vi "Framework Page.vi"(8 "error in (no error)":errorcluster, 11 "Node Ptr":T1 format="%.0x") -> (0 "error out":errorcluster)   [LabVIEW 2017, in "DSF System Explorer.lvlib"]
uses:
  DSF System Explorer.lvlib
  <vilib>/NI Veristand/Custom Device API/Custom Device Item Ref.ctl
  <vilib>/NI Veristand/Custom Device API/Custom Device API.lvlib
  Shared/DSF Shared.lvlib
  Data Viewer.lvlibp
panel:
  in  "New":bool
  in  "Version":string
  in  "Export":bool
  in  "Debug Mode":bool
  in  "Launch Data Viewer":bool
  in  "Server Frequency":dbl=20.0 format="%.0f Hz"
  in  "Enable Data Server":bool
  in  "Show Dialog on Error":bool
  in  "Show Threads":bool
  in  "Infinite FIFO Timeouts":bool
  in  "Measure Durations":bool
  in  "Measure Period":bool
  in  "Import":bool
  in  "View Configuration":bool
  in  "Header":cluster{"Section Name":string}={"Section Name"="Data Sharing Framework"}
  # "Debug Options"
  # "Measurement Options"
  # "Data Server Options"
  # "All Targets"
  # "All Targets"
  # "All Targets"
  # "Windows Only"
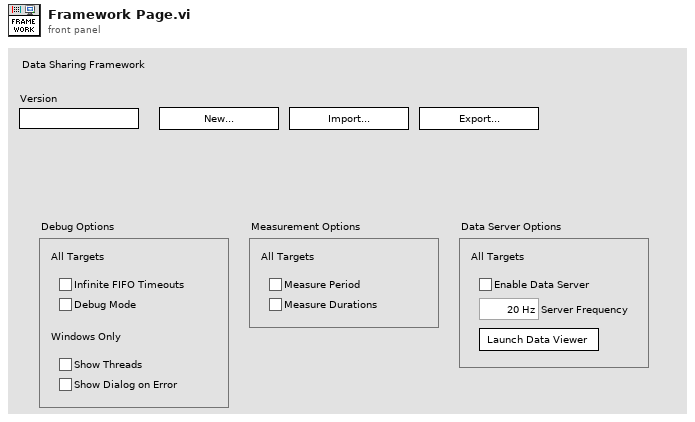
[diagram p1: front panel]
types:
  T1 = typedef "Custom Device API.lvlib/Custom Device Item Ref.ctl" = u64
  T2 = typedef "DSF Core.lvlibp/Framework.lvclass/Framework Options.ctl" = cluster{"FIFO Options":T3, "Thread Options":T4, "Plugin Options":T5, "Performance Options":T6, "Data Server Options":T7}
  T3 = typedef "DSF Core.lvlibp/Framework.lvclass/DSF FIFO Options.ctl" = cluster{"Infinite Timeouts":bool}
  T4 = typedef "DSF Core.lvlibp/Thread.lvclass/Thread Options.ctl" = cluster{"Show FP On Call":bool, "Close FP After Call":bool, "Allow Debugging":bool}
  T5 = typedef "DSF Core.lvlibp/Framework.lvclass/DSF Plugin Options.ctl" = cluster{"Default Components":bool}
  T6 = typedef "DSF Core.lvlibp/DSF Performance Options.ctl" = cluster{"Measure Period":bool, "Measure Rx/Tx Duration":bool}
  T7 = typedef "DSF Core.lvlibp/Framework.lvclass/Data Server Options.ctl" = cluster{"Enable Data Server":bool, "Period":u32}
  T8 = typedef "DSF Core.lvlibp/DSF Version Info.ctl" = cluster{"major":u32, "minor":u32, "fix":u32, "build":string}
  T9 = typedef "Custom Device API.lvlib/Custom Device Commands.ctl" = enum16{"Default", "Item renamed", "Shutdown", "Dynamic button pressed"}
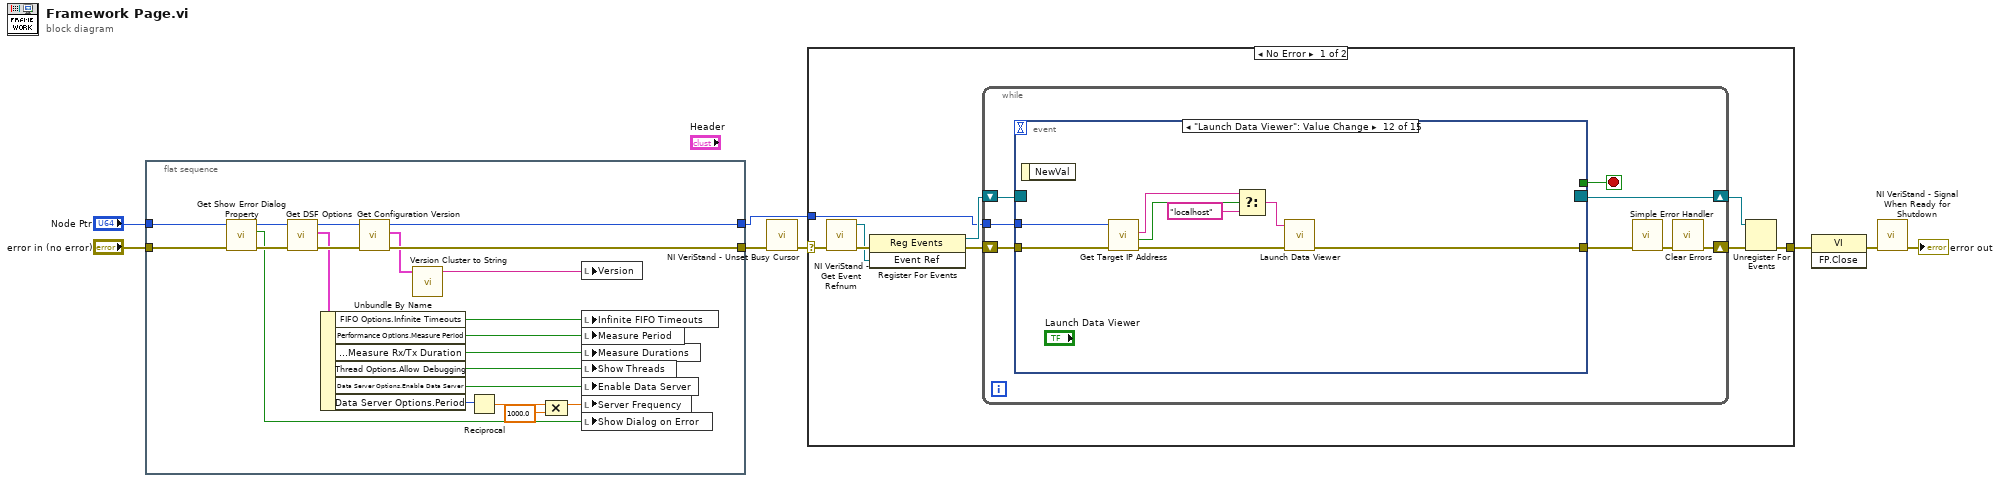
[diagram p0: block diagram]
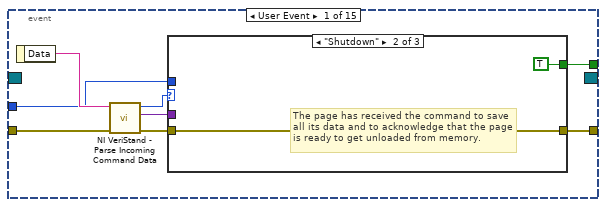
[diagram p2: hidden frame]
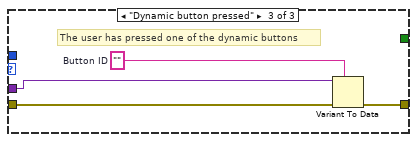
[diagram p4: hidden frame]
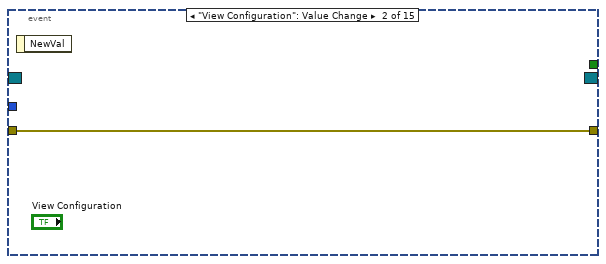
[diagram p5: hidden frame]
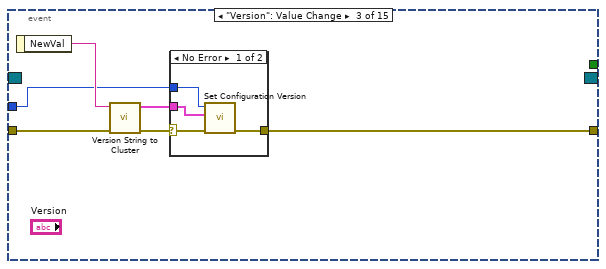
[diagram p6: hidden frame]
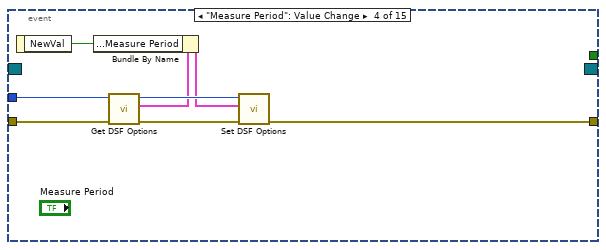
[diagram p8: hidden frame]
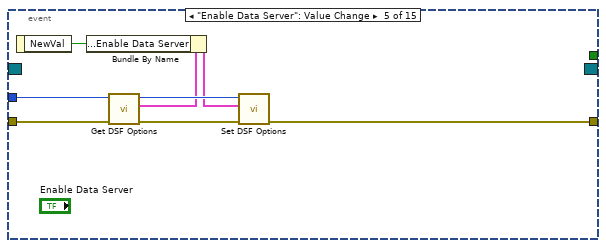
[diagram p9: hidden frame]
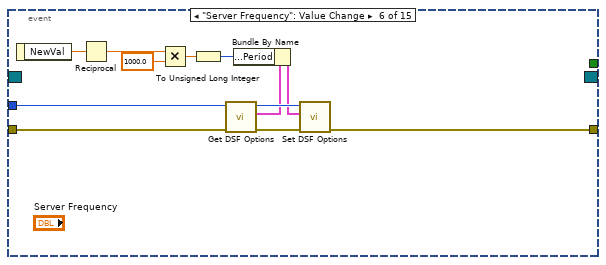
[diagram p10: hidden frame]
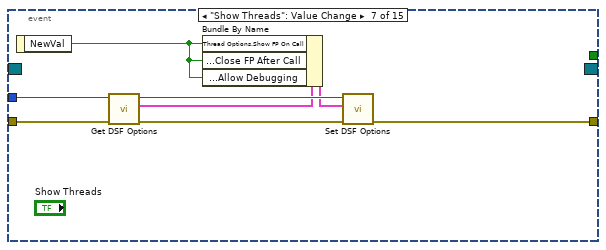
[diagram p11: hidden frame]
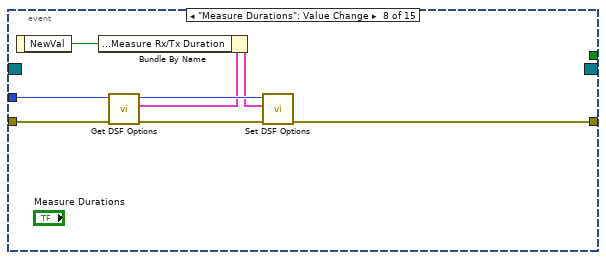
[diagram p12: hidden frame]
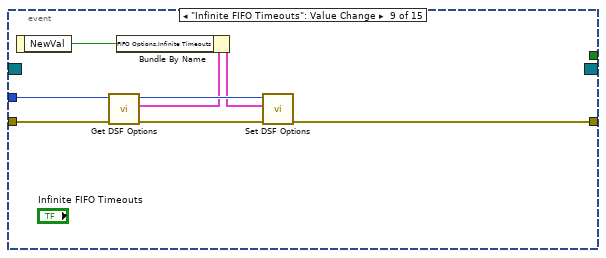
[diagram p13: hidden frame]
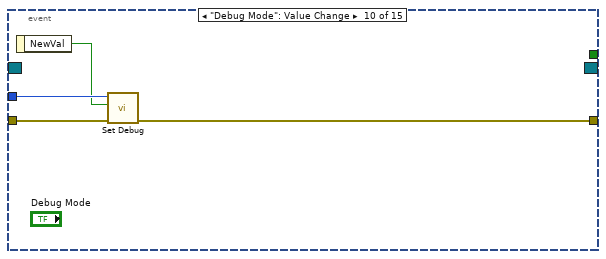
[diagram p14: hidden frame]
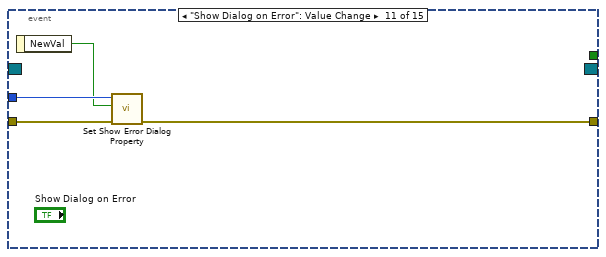
[diagram p15: hidden frame]
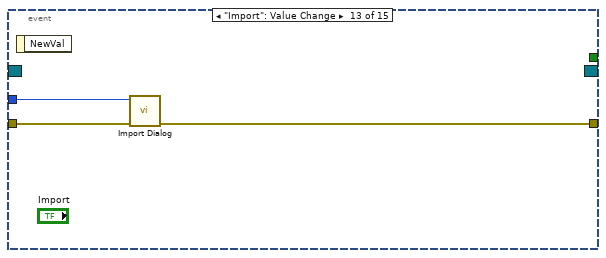
[diagram p16: hidden frame]
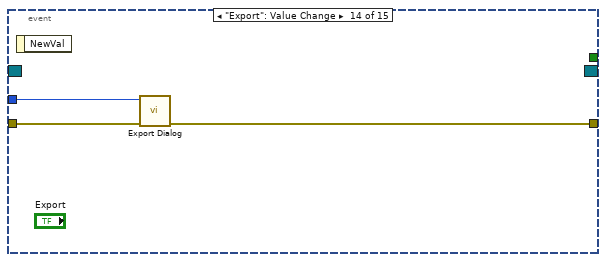
[diagram p17: hidden frame]
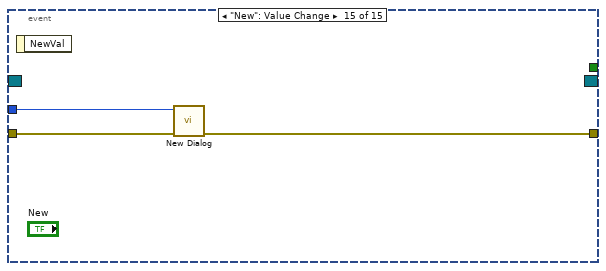
[diagram p18: hidden frame]
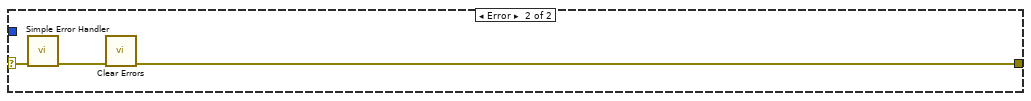
[diagram p19: hidden frame]
diagram:
  n1 = flat-sequence "Initialization code" {
    tunnel: "error in (no error)" -> [w9]
    tunnel: "Node Ptr" -> [w10]
    tunnel: [w14] -> w4
    tunnel: [w13] -> w1
    frame #0 {
      n2 = call "Get Show Error Dialog Property.vi"("error in (no error)"=w9, "Item Ref in"=w10) -> ("error out"=w24:errorcluster, "show error dialog"=w18:bool, "Item Ref out"=w25:T1)  [unwired: 7 in]
      n3 = call "Get DSF Options.vi"("error in (no error)"=w24, "Item Ref in"=w25) -> ("error out"=w17:errorcluster, "options"=w15:T2, "Item Ref out"=w16:T1)  [unwired: 7 in]
      n4 = Unbundle By Name(w15) -> ("FIFO Options.Infinite Timeouts"=w29:bool, "Performance Options.Measure Period"=w28:bool, "Performance Options.Measure Rx/Tx Duration"=w27:bool, "Thread Options.Allow Debugging"=w26:bool, "Data Server Options.Enable Data Server"=w23:bool, "Data Server Options.Period"=w22:u32)
      n5 = call "Get Configuration Version.vi"("error in (no error)"=w17, "Item Ref in"=w16) -> ("error out"=w14:errorcluster, "version"=w12:T8, "Item Ref out"=w13:T1)  [unwired: 7 in]
      n6 = call "Version Cluster to String.vi"("version"=w12) -> ("version string"=w11:string)  [unwired: 9 in, 1 out]
      n7 = Reciprocal(x=w22) -> (1/x=w21:dbl)
      n8 = Compound Arithmetic op=MULTIPLY(w21, 1000.0 ("y")) -> (w20:dbl)
      n9 = local write "Version"(w11) -> ()
      n10 = local write "Infinite FIFO Timeouts"(w29) -> ()
      n11 = local write "Measure Period"(w28) -> ()
      n12 = local write "Measure Durations"(w27) -> ()
      n13 = local write "Show Threads"(w26) -> ()
      n14 = local write "Enable Data Server"(w23) -> ()
      n15 = local write "Server Frequency"(w20) -> ()
      n16 = local write "Show Dialog on Error"(w18) -> ()
    }
  }
  n17 = call <vilib>:"NI VeriStand - Unset Busy Cursor.vi"("error in (no error)"=w4) -> ("error out"=w3:errorcluster)  [unwired: 10 out]
  n18 = case shown="No Error" w3 {
    selector: w3 -> [w30 w153]
    tunnel: [w35 w151] -> w8
    tunnel: w1 -> [w31 _]
    frame No Error {
      n19 = call <vilib>:"NI VeriStand - Get Event Refnum.vi"("error in (no error)"=w30) -> ("error out"=w38:errorcluster, "Event Ref"=w34:refnum<user-event>)  [unwired: 9 out]
      n20 = register-events(error in=w38, w34) -> (reference out=w32:refnum<event-registration>, error out=w33:errorcluster)  [unwired: 1 in]
      n21 = while {
        tunnel: w31 -> [w42]
        shift-right: [w39] -> w36
        shift-left: w33 -> [w45]
        shift-right: [w46] -> w37
        shift-left: w32 -> [w44]
        stop <- w43 stop-if-true
        n22 = event shown="[11] \"Launch Data Viewer\": Value Change" {
          selector: w44 -> [_ _ _ _ _ _ _ _ _ _ _ _ _ _ _]
          dyn-events: [_ _ _ _ _ _ _ _ _ _ _ _ _ _ _] -> w46
          timeout: _ -> [_ _ _ _ _ _ _ _ _ _ _ _ _ _ _]
          tunnel: w45 -> [w54 w62 w68 w79 w87 w100 w108 w115 w123 w129 w133 w141 w144 w147 w150]
          tunnel: [w50 _ _ _ _ _ _ _ _ _ _ _ _ _ _] -> w43
          tunnel: [w49 w62 w65 w76 w84 w98 w105 w112 w120 w126 w131 w138 w142 w145 w148] -> w41
          tunnel: w42 -> [w48 _ w63 w81 w89 w101 w109 w117 w125 w128 w132 w140 w143 w146 w149]
          event User Event {
            n23 = event-data() -> ("Data"=w53:string)  [unwired: 1 out]
            n24 = call <vilib>:"NI VeriStand - Parse Incoming Command Data.vi"("error in (no error)"=w54, "Incoming data"=w53) -> ("error out"=w52:errorcluster, "Outgoing data"=w47:variant, "Action"=w51:T9)  [unwired: 7 out]
            n25 = case shown="\"Shutdown\"" w51 {
              tunnel: w52 -> [w55 w56 w61]
              tunnel: [_ TRUE _] -> w50
              tunnel: [w55 w56 w58] -> w49
              tunnel: w48 -> [_ _ _]
              tunnel: w47 -> [_ _ w60]
              frame "Default", Default {
              }
              frame "Shutdown" {
                # "The page has received the command to save all its data and to acknowledge that the page is ready to get unloaded from memory."
              }
              frame "Dynamic button pressed" {
                w59 = ""  # Button ID
                # "The user has pressed one of the dynamic buttons"
                n26 = Variant To Data(error in=w61, type=w59, Variant=w60) -> (error out=w58:errorcluster)  [unwired: 1 out]
              }
            }
          }
          event "View Configuration": Value Change {
            n27 = event-data() -> ()  [unwired: 2 out]
          }
          event "Version": Value Change {
            n28 = event-data() -> ("NewVal"=w67:string)  [unwired: 1 out]
            n29 = call "Version String to Cluster.vi"("error in (no error)"=w68, "version string"=w67) -> ("error out"=w66:errorcluster, "version"=w64:T8)  [unwired: 8 in]
            n30 = case shown="No Error" w66 {
              selector: w66 -> [w72 w73]
              tunnel: [w69 w73] -> w65
              tunnel: w64 -> [w71 _]
              tunnel: w63 -> [w70 _]
              frame No Error {
                n31 = call "Set Configuration Version.vi"("error in (no error)"=w72, "version"=w71, "Item Ref in"=w70) -> ("error out"=w69:errorcluster)  [unwired: 7 in, 1 out]
              }
              frame Error {
              }
            }
          }
          event "Measure Period": Value Change {
            n32 = event-data() -> ("NewVal"=w80:bool)  [unwired: 1 out]
            n33 = call "Get DSF Options.vi"("error in (no error)"=w79, "Item Ref in"=w81) -> ("error out"=w77:errorcluster, "options"=w74:T2, "Item Ref out"=w78:T1)  [unwired: 7 in]
            n34 = Bundle By Name(cluster=w74, "Performance Options.Measure Period"=w80) -> (w75:T2)
            n35 = call "Set DSF Options.vi"("error in (no error)"=w77, "options"=w75, "Item Ref in"=w78) -> ("error out"=w76:errorcluster)  [unwired: 7 in, 1 out]
          }
          event "Enable Data Server": Value Change {
            n36 = event-data() -> ("NewVal"=w88:bool)  [unwired: 1 out]
            n37 = call "Get DSF Options.vi"("error in (no error)"=w87, "Item Ref in"=w89) -> ("error out"=w85:errorcluster, "options"=w82:T2, "Item Ref out"=w86:T1)  [unwired: 7 in]
            n38 = Bundle By Name(cluster=w82, "Data Server Options.Enable Data Server"=w88) -> (w83:T2)
            n39 = call "Set DSF Options.vi"("error in (no error)"=w85, "options"=w83, "Item Ref in"=w86) -> ("error out"=w84:errorcluster)  [unwired: 7 in, 1 out]
          }
          event "Server Frequency": Value Change {
            n40 = event-data() -> ("NewVal"=w95:dbl)  [unwired: 1 out]
            n41 = Reciprocal(x=w95) -> (1/x=w91:dbl)
            n42 = Multiply(x=w91, y=1000.0) -> (x*y=w92:dbl)
            n43 = To Unsigned Long Integer(number=w92) -> (unsigned 32bit integer=w94:u32)
            n44 = call "Get DSF Options.vi"("error in (no error)"=w100, "Item Ref in"=w101) -> ("error out"=w93:errorcluster, "options"=w96:T2, "Item Ref out"=w99:T1)  [unwired: 7 in]
            n45 = Bundle By Name(cluster=w96, "Data Server Options.Period"=w94) -> (w97:T2)
            n46 = call "Set DSF Options.vi"("error in (no error)"=w93, "options"=w97, "Item Ref in"=w99) -> ("error out"=w98:errorcluster)  [unwired: 7 in, 1 out]
          }
          event "Show Threads": Value Change {
            n47 = event-data() -> ("NewVal"=w102:bool)  [unwired: 1 out]
            n48 = call "Get DSF Options.vi"("error in (no error)"=w108, "Item Ref in"=w109) -> ("error out"=w106:errorcluster, "options"=w103:T2, "Item Ref out"=w107:T1)  [unwired: 7 in]
            n49 = Bundle By Name(cluster=w103, "Thread Options.Show FP On Call"=w102, "Thread Options.Close FP After Call"=w102, "Thread Options.Allow Debugging"=w102) -> (w104:T2)
            n50 = call "Set DSF Options.vi"("error in (no error)"=w106, "options"=w104, "Item Ref in"=w107) -> ("error out"=w105:errorcluster)  [unwired: 7 in, 1 out]
          }
          event "Measure Durations": Value Change {
            n51 = event-data() -> ("NewVal"=w116:bool)  [unwired: 1 out]
            n52 = call "Get DSF Options.vi"("error in (no error)"=w115, "Item Ref in"=w117) -> ("error out"=w113:errorcluster, "options"=w110:T2, "Item Ref out"=w114:T1)  [unwired: 7 in]
            n53 = Bundle By Name(cluster=w110, "Performance Options.Measure Rx/Tx Duration"=w116) -> (w111:T2)
            n54 = call "Set DSF Options.vi"("error in (no error)"=w113, "options"=w111, "Item Ref in"=w114) -> ("error out"=w112:errorcluster)  [unwired: 7 in, 1 out]
          }
          event "Infinite FIFO Timeouts": Value Change {
            n55 = event-data() -> ("NewVal"=w124:bool)  [unwired: 1 out]
            n56 = call "Get DSF Options.vi"("error in (no error)"=w123, "Item Ref in"=w125) -> ("error out"=w121:errorcluster, "options"=w118:T2, "Item Ref out"=w122:T1)  [unwired: 7 in]
            n57 = Bundle By Name(cluster=w118, "FIFO Options.Infinite Timeouts"=w124) -> (w119:T2)
            n58 = call "Set DSF Options.vi"("error in (no error)"=w121, "options"=w119, "Item Ref in"=w122) -> ("error out"=w120:errorcluster)  [unwired: 7 in, 1 out]
          }
          event "Debug Mode": Value Change {
            n59 = event-data() -> ("NewVal"=w127:bool)  [unwired: 1 out]
            n60 = call "Set Debug.vi"("error in (no error)"=w129, "debug"=w127, "Item Ref in"=w128) -> ("error out"=w126:errorcluster)  [unwired: 7 in, 1 out]
          }
          event "Show Dialog on Error": Value Change {
            n61 = event-data() -> ("NewVal"=w130:bool)  [unwired: 1 out]
            n62 = call "Set Show Error Dialog Property.vi"("error in (no error)"=w133, "show error dialog"=w130, "Item Ref in"=w132) -> ("error out"=w131:errorcluster)  [unwired: 7 in, 1 out]
          }
          event "Launch Data Viewer": Value Change {
            n63 = event-data() -> ()  [unwired: 2 out]
            n64 = call "Get Target IP Address.vi"("error in (no error)"=w141, "Item Ref in"=w140) -> ("error out"=w139:errorcluster, "found"=w136:bool, "target address"=w137:string)  [unwired: 6 in, 1 out]
            n65 = Select(t=w137, s=w136, f="localhost") -> (s? t:f=w134:string)
            n66 = call "Launch Data Viewer.vi"("error in (no error)"=w139, "Server IP Address (localhost)"=w134) -> ("error out"=w138:errorcluster)  [unwired: 9 in]
          }
          event "Import": Value Change {
            n67 = event-data() -> ()  [unwired: 2 out]
            n68 = call "Import Dialog.vi"("error in (no error)"=w144, "Item Ref in"=w143) -> ("error out"=w142:errorcluster)  [unwired: 8 in, 1 out]
          }
          event "Export": Value Change {
            n69 = event-data() -> ()  [unwired: 2 out]
            n70 = call "Export Dialog.vi"("error in (no error)"=w147, "Item Ref in"=w146) -> ("error out"=w145:errorcluster)  [unwired: 8 in, 1 out]
          }
          event "New": Value Change {
            n71 = event-data() -> ()  [unwired: 2 out]
            n72 = call "New Dialog.vi"("error in (no error)"=w150, "Item Ref in"=w149) -> ("error out"=w148:errorcluster)  [unwired: 8 in, 1 out]
          }
        }
        n73 = call <vilib>:"Simple Error Handler.vi"("error in (no error)"=w41) -> ("error out"=w40:errorcluster)  [unwired: 1 in, 7 out]
        n74 = call <vilib>:"Clear Errors.vi"("error in (no error)"=w40) -> ("error out"=w39:errorcluster)  [unwired: 1 in, 5 out]
      }
      n75 = Unregister For Events(event registration refnum=w37, error in=w36) -> (error out=w35:errorcluster)
    }
    frame Error {
      n76 = call <vilib>:"Simple Error Handler.vi"("error in (no error)"=w153) -> ("error out"=w152:errorcluster)  [unwired: 1 in, 7 out]
      n77 = call <vilib>:"Clear Errors.vi"("error in (no error)"=w152) -> ("error out"=w151:errorcluster)  [unwired: 1 in, 5 out]
    }
  }
  n78 = invoke class="VI" method="FP.Close"(error in=w8) -> (error out=w7:errorcluster)  [unwired: 2 in, 2 out]
  n79 = call <vilib>:"NI VeriStand - Signal When Ready for Shutdown.vi"("error in (no error)"=w7) -> ("error out"=→"error out":errorcluster)  [unwired: 10 out]
